vi "factorialofanumber.vi"(1 "n":dbl) -> (0 "n!":dbl)   [LabVIEW 2024]
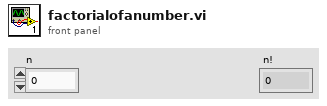
[diagram p1: front panel]
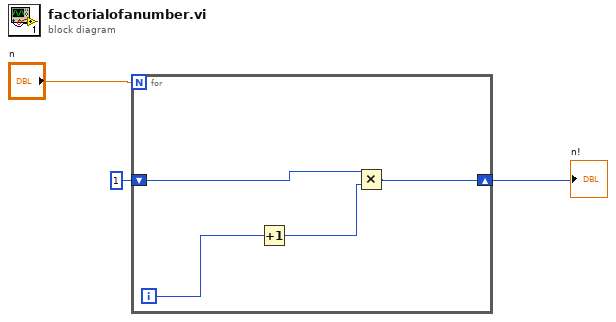
[diagram p0: block diagram]
diagram:
  n1 = for {
    N: "n" -> [_]
    shift-right: [w7] -> w2
    shift-left: 1 -> [w6]
    i -> [w5]
    n2 = Increment(x=w5) -> (x+1=w4:i32)
    n3 = Multiply(x=w6, y=w4) -> (x*y=w7:i32)
  }
  "n!" <- w2
